vi "Run Power Spectrum Density.vi"(6 "Channel Name":string, 8 "Percentage":dbl, 9 "Data Valid":bool, 10 "Signal":waveform(dbl)={"t0"=timestamp(0 s since 1904-01-01), "dt"=0.0, "Y"=[]}, 11 "Data":T1={"First Time"=FALSE, "Show PSD Window"=FALSE, "Show PSD Window Clicked"=FALSE, "Export mode"=0, "Window"=1, "dB"=FALSE, "Averaging parameters"={"averaging mode"=enum."No averaging", "weighting mode"=enum."Exponential", "number of averages"=10}, "Window parameter"=nan, "Number of Samples"=1000, "PSD VI Ref"=refnum} {"Averaging parameters"."number of averages" min=1; "Window" items=["Rectangle"=0, "Hanning"=1, "Hamming"=2, "Blackman-Harris"=3, "Exact Blackman"=4, "Blackman"=5, "Flat Top"=6, "4 Term B-Harris "=7, "7 Term B-Harris"=8, "Low Sidelobe"=9, "Blackman Nuttall"=11, "Triangle"=30, "Bartlett-Hanning"=31, "Bohman"=32, "Parzen"=33, "Welch"=34, "Kaiser"=60, "Dolph-Chebyshev"=61, "Gaussian"=62]; "Export mode" items=["Power Spectrum", "Power Spectral Density"]}) -> (3 "Data out":T1={"First Time"=FALSE, "Show PSD Window"=FALSE, "Show PSD Window Clicked"=FALSE, "Export mode"=0, "Window"=1, "dB"=FALSE, "Averaging parameters"={"averaging mode"=enum."No averaging", "weighting mode"=enum."Exponential", "number of averages"=10}, "Window parameter"=nan, "Number of Samples"=1000, "PSD VI Ref"=refnum} {"Averaging parameters"."number of averages" min=1; "Window" items=["Rectangle"=0, "Hanning"=1, "Hamming"=2, "Blackman-Harris"=3, "Exact Blackman"=4, "Blackman"=5, "Flat Top"=6, "4 Term B-Harris "=7, "7 Term B-Harris"=8, "Low Sidelobe"=9, "Blackman Nuttall"=11, "Triangle"=30, "Bartlett-Hanning"=31, "Bohman"=32, "Parzen"=33, "Welch"=34, "Kaiser"=60, "Dolph-Chebyshev"=61, "Gaussian"=62]; "Export mode" items=["Power Spectrum", "Power Spectral Density"]})   [LabVIEW 2023, in "Power Spectrum Density.lvlib" / "Power Spectrum Density.lvclass"]
uses:
  Power Spectrum Density.lvclass
  Power Spectrum Density.lvclass/Power Spectrum Density.ctl
  <vilib>/measure/maspectr.llb/Power Spectrum and PSD Export Mode.ctl
  <vilib>/measure/NI_MAPro.lvlib
  <vilib>/Analysis/4window.llb/windowTd.ctl
  <vilib>/Analysis/NI_AALPro.lvlib
  Power Spectrum Density Data.ctl
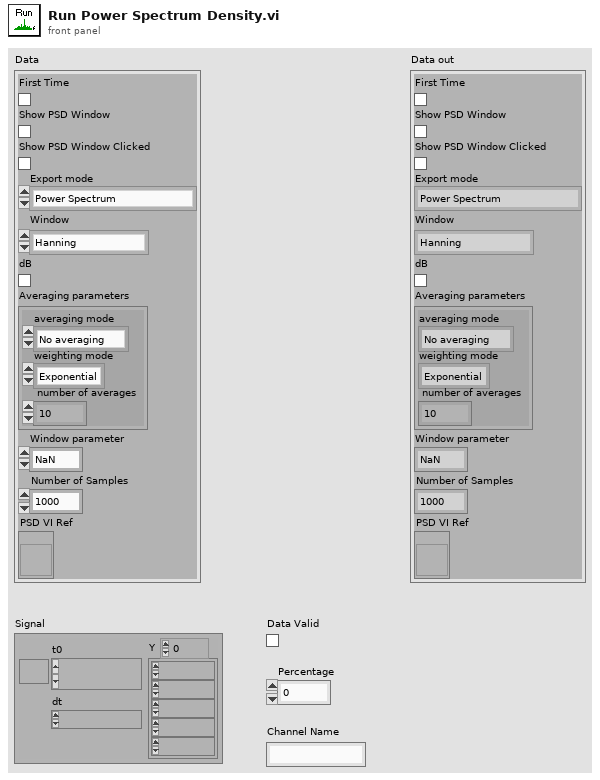
[diagram p1: front panel]
types:
  T1 = typedef "Power Spectrum Density.lvlib/Power Spectrum Density.lvclass/Power Spectrum Density Data.ctl" = cluster{"First Time":bool, "Show PSD Window":bool, "Show PSD Window Clicked":bool, "Export mode":T2, "Window":T3, "dB":bool, "Averaging parameters":cluster{"averaging mode":enum16{"No averaging", "Vector averaging", "RMS averaging", "Peak hold"}, "weighting mode":enum16{"Linear", "Exponential"}, "number of averages":u32}, "Window parameter":dbl, "Number of Samples":i32, "PSD VI Ref":refnum<vi>}
  T2 = typedef "NI_MAPro.lvlib/Power Spectrum and PSD Export Mode.ctl" = u16
  T3 = typedef "NI_AALPro.lvlib/windowTd.ctl" = u32
  T4 = cluster{"averaging mode":enum16{"No averaging", "Vector averaging", "RMS averaging", "Peak hold"}, "weighting mode":enum16{"Linear", "Exponential"}, "number of averages":u32}
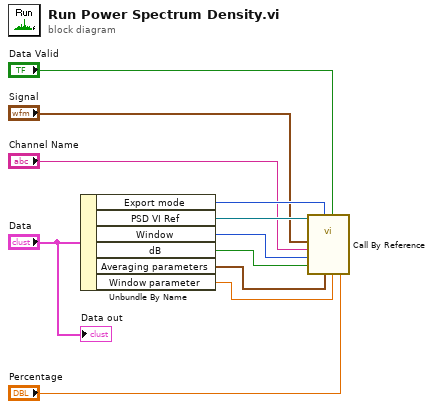
[diagram p0: block diagram]
diagram:
  n1 = Unbundle By Name("Data") -> ("Export mode"=w11:T2, "PSD VI Ref"=w10:refnum<vi>, "Window"=w7:T3, "dB"=w6:bool, "Averaging parameters"=w5:T4, "Window parameter"=w4:dbl)
  n2 = call-by-ref "?"(reference=w10, "Percentage"="Percentage", "window parameter"=w4, "Data Valid"="Data Valid", "averaging parameters"=w5, "export mode"=w11, "dB"=w6, "window"=w7, "Channel Name"="Channel Name", "Signal"="Signal") -> ()  [unwired: 4 in, 2 out]
  "Data out" <- "Data"
